vi "Constant--default font.vi"() -> (1 "Font size":u32, 2 "Font name":string)   [LabVIEW 2020, in "status_text_indicator.lvlib"]
uses:
  Status_Text_Indicator.lvlib
panel:
  # "Development\ncontrols/indicators useful for development and testing, but which are not outputs of the VI"
  # "Input\nInputs to the VI"
  # "Output\nOutputs of the VI"
  # "Description\n\nBlank VI with error handling case. \n\nSummarize the use of this VI in this space."
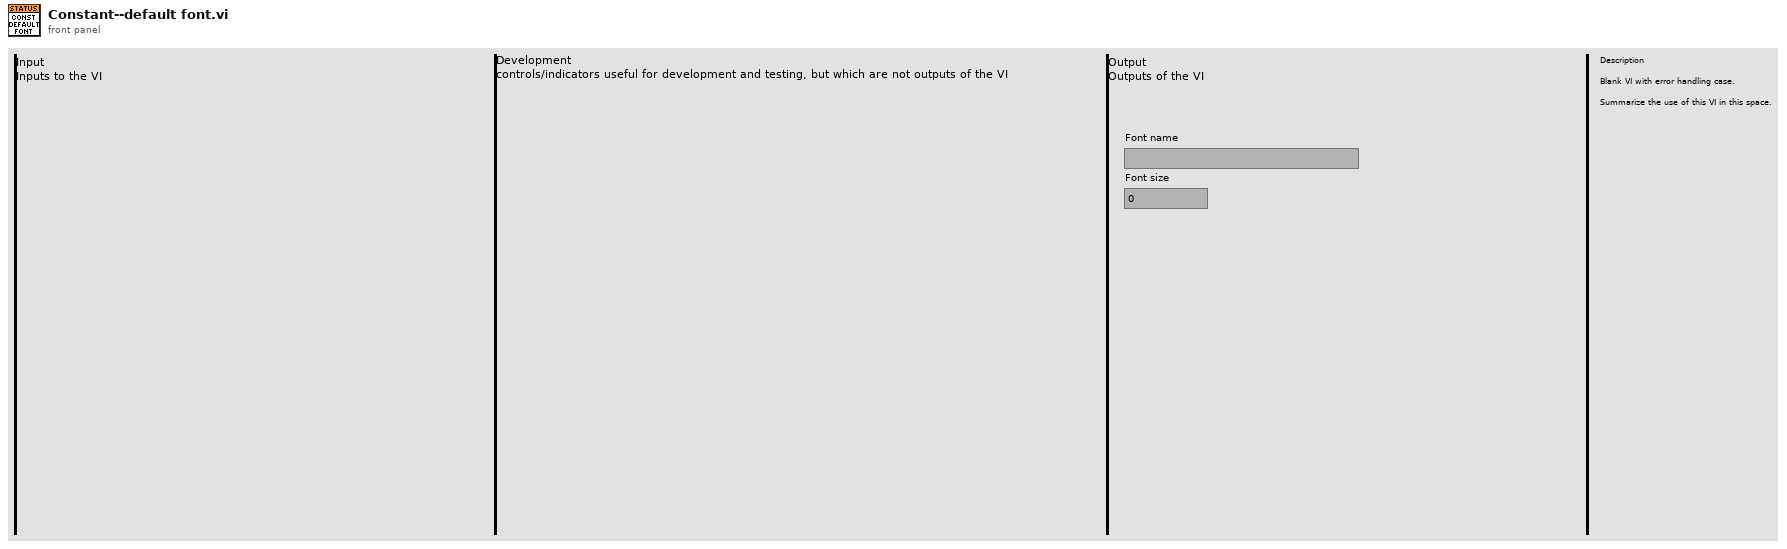
[diagram p1: front panel]
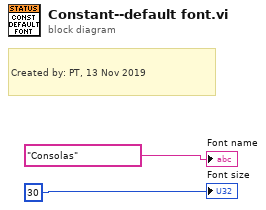
[diagram p0: block diagram]
diagram:
  # "Created by: PT, 13 Nov 2019"
  "Font name" <- "Consolas" ("Font:Name")
  "Font size" <- u32 30 ("Text.Font:Size (Dflt=15pt)")
